vi "Correct Abs Time of FPGA.vi"(8 "error in":errorcluster, 9 "FTE Terminal":tag="/Dev1/PXI_Trig7", 10 "IVI Refnum in":refnum<k15>, 11 "Session In":refnum<k20>) -> (0 "error out":errorcluster, 2 "IVI Refnum out":refnum<k15>, 3 "Session Out":refnum<k20>)   [LabVIEW 2016]
uses:
  <vilib>/Utility/error.llb/Error Cluster From Error Code.vi
  <vilib>/rvi/errors/niLvFpgaAdjustHostInterfaceError.vi
  <vilib>/rvi/interface/nirviReadWriteControl/nirviReadWriteControl.xnode
  <vilib>/rvi/interface/Simulation/niFpgaSimulationCallBeginRW.vi
  NiFpgaLv.dll
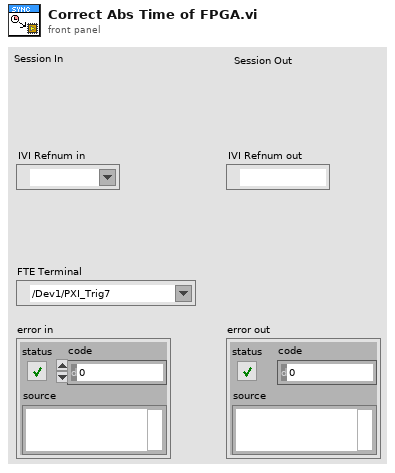
[diagram p1: front panel]
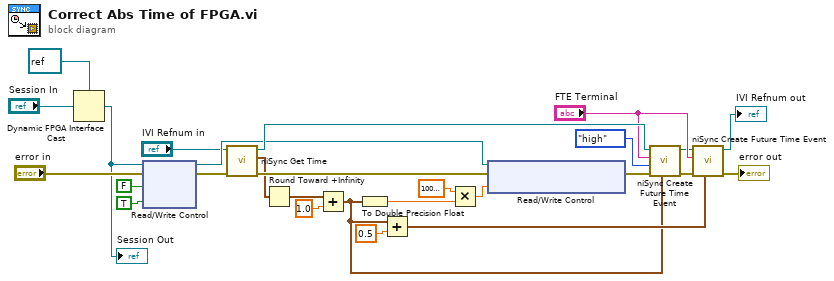
[diagram p0: block diagram]
diagram:
  n1 = Dynamic FPGA Interface Cast(Session In=refnum<k20> refnum ("Type"), Type="Session In") -> (Session Out=w2:refnum<k20>)
  "Session Out" <- w2
  n2 = xnode "Read/Write Control"("FPGA VI Reference In"=w2, "error in"="error in", "Lock"=FALSE, "Lock"=TRUE) -> ("FPGA VI Reference Out"=w23:refnum<k20>, "error out"=w26:errorcluster)
  n3 = call <instrlib>:"niSync Get Time.vi"("error in (no error)"=w26, "instrument handle"="IVI Refnum in") -> ("error out"=w7:errorcluster, "time"=w4:timestamp, "instrument handle out"=w27:refnum<k15>)  [unwired: 5 in]
  n4 = Round Toward +Infinity(x=w4) -> (ceil(x): smallest int >= x=w5:timestamp)
  n5 = Add(x=w5, y=1.0) -> (x+y=w15:timestamp)
  n6 = To Double Precision Float(number=w15) -> (double precision float=w20:dbl)
  n7 = Add(x=w15, y=0.5) -> (x+y=w17:timestamp)
  n8 = Multiply(x=1000000000.0, y=w20) -> (x*y=w19:dbl)
  n9 = xnode "Read/Write Control"("FPGA VI Reference In"=w23, "error in"=w7, "Sync Counter Load Val"=w19) -> ("error out"=w8:errorcluster)  [unwired: 1 out]
  n10 = call <instrlib>:"niSync Create Future Time Event.vi"("time"=w15, "error in (no error)"=w8, "output level"=enum32{"low", "high"}."high", "terminal"="FTE Terminal", "instrument handle"=w27) -> ("error out"=w12:errorcluster, "instrument handle out"=w11:refnum<k15>)  [unwired: 4 in]
  n11 = call <instrlib>:"niSync Create Future Time Event.vi"("time"=w17, "error in (no error)"=w12, "terminal"="FTE Terminal", "instrument handle"=w11) -> ("error out"=→"error out":errorcluster, "instrument handle out"=→"IVI Refnum out":refnum<k15>)  [unwired: 5 in]
